vi "GS_Write_Config.vi"(4 "error in (no error)":errorcluster, 7 "Config Refnum":T1) -> (0 "error out":errorcluster, 3 "refnum out":T1)   [LabVIEW 2015]
uses:
  <vilib>/Utility/config.llb/Config Data RefNum.ctl
  GSCS Scripting/Utils/GSP_Wavelength_Global.vi
  <vilib>/Utility/config.llb/Write Key (Double).vi
  <vilib>/Utility/config.llb/NI_LVConfig.lvlib
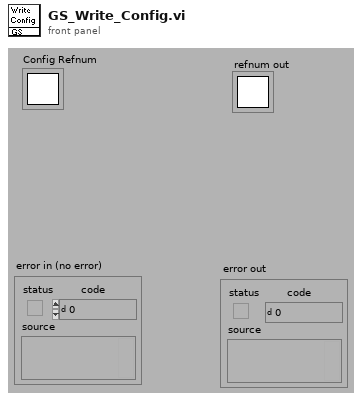
[diagram p1: front panel]
types:
  T1 = typedef "NI_LVConfig.lvlib/Config Data RefNum.ctl" = refnum<k1>
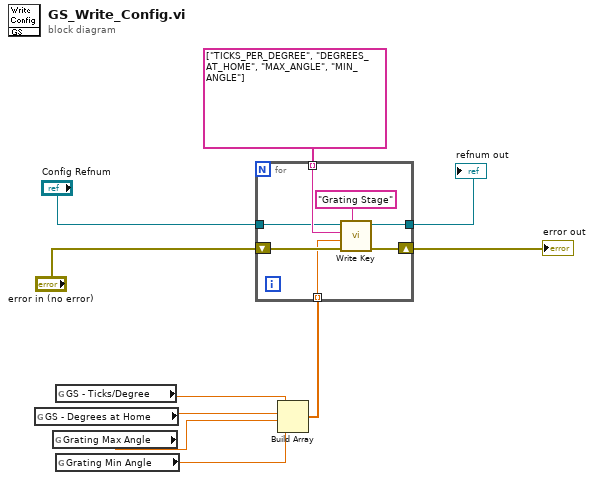
[diagram p0: block diagram]
diagram:
  n1 = global read "GSP_Wavelength_Global.vi" "GS - Degrees at Home"() -> (w7:dbl)
  n2 = global read "GSP_Wavelength_Global.vi" "Grating Max Angle"() -> (w2:dbl)
  n3 = global read "GSP_Wavelength_Global.vi" "GS - Ticks/Degree"() -> (w8:dbl)
  n4 = global read "GSP_Wavelength_Global.vi" "Grating Min Angle"() -> (w1:dbl)
  n5 = Build Array(w8, w7, w2, w1) -> (w10:dbl[])
  n6 = for {
    shift-right: [w15] -> w5
    shift-left: "error in (no error)" -> [w17]
    tunnel: [w14] -> w6
    tunnel: w10 -> [w13] mode=indexing
    tunnel: string[] ["TICKS_PER_DEGREE", "DEGREES_AT_HOME", "MAX_ANGLE", "MIN_ANGLE"] -> [w12] mode=indexing
    tunnel: "Config Refnum" -> [w11]
    n7 = call-poly <vilib>:"Write Key.vi"("section"="Grating Stage", "error in (no error)"=w17, "value"=w13, "key"=w12, "refnum"=w11) -> ("error out"=w15:errorcluster, "refnum out"=w14:T1)  [unwired: 4 in, 1 out]
  }
  "error out" <- w5
  "refnum out" <- w6
